vi "I2C.WriteString.vi"(5 "I2C Address":u16 format="%x", 7 "I2C Register":u16 format="%x", 8 "error in":errorcluster, 9 "Append NULL Char?":bool, 10 "I2C Write Data":string, 11 "comport in":refnum<visa-resource-name>) -> (0 "error out":errorcluster, 1 "WrittenBytes":i32, 3 "comport out":refnum<visa-resource-name>)   [LabVIEW 2020, in "FirmataClient.lvlib"]
doc: "Transmit a string to the UUT for a target I2C device running on its board"
uses:
  FirmataClient.lvlib
panel:
  in  "DownloadChunkSize":u8=30
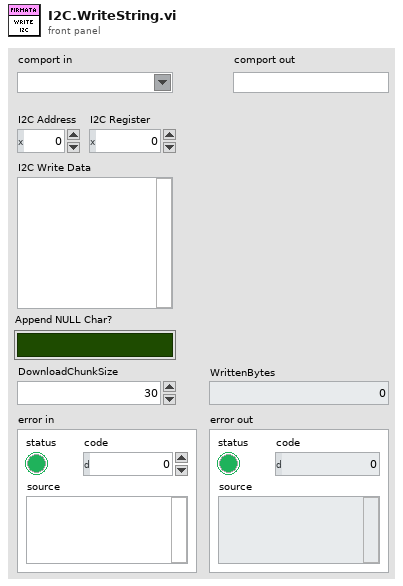
[diagram p1: front panel]
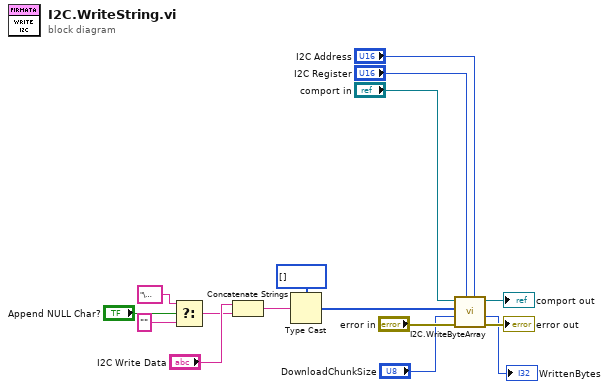
[diagram p0: block diagram]
diagram:
  n1 = Select(t="\u0000", s="Append NULL Char?", f="") -> (s? t:f=w15:string)
  n2 = Concatenate Strings("I2C Write Data", w15) -> (w5:string)
  n3 = Type Cast(type=u8[] [] ("I2C Write Data"), x=w5) -> (*(type *) &x=w1:u8[])
  n4 = call "I2C.WriteByteArray.vi"("I2C Address"="I2C Address", "I2C Register"="I2C Register", "error in"="error in", "DownloadChunkSize"="DownloadChunkSize", "I2C Write Data"=w1, "comport in"="comport in") -> ("error out"=→"error out":errorcluster, "WrittenBytes"=→"WrittenBytes":i32, "comport out"=→"comport out":refnum<visa-resource-name>)  [unwired: 3 in]
